vi "detectPulse.vi"(1 "filteredECG":waveform(dbl)) -> (0 "PulseBPM":dbl)   [LabVIEW 2023]
uses:
  <vilib>/measure/mamon.llb/Waveform Peak Detection for 1 Chan.vi
  <vilib>/measure/NI_MAPro.lvlib
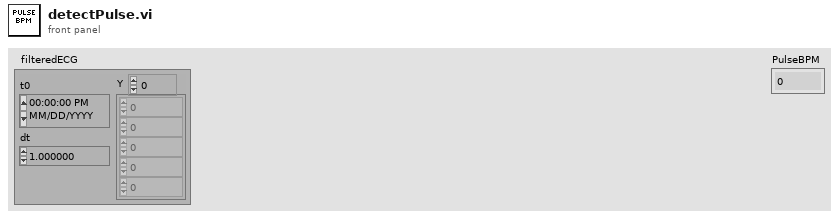
[diagram p1: front panel]
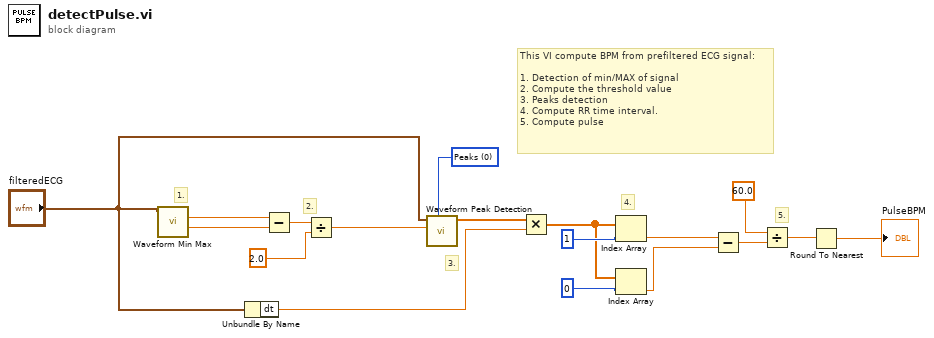
[diagram p0: block diagram]
diagram:
  w1 = u16 0 items=["Peaks", "Valleys"] ("peaks/valleys")
  # "5."
  # "This VI compute BPM from prefiltered ECG signal:\n\n1. Detection of min/MAX of signal\n2. Compute the threshold value\n3. Peaks detection\n4. Compute RR time interval.\n5. Compute pulse"
  # "4."
  # "3."
  # "2."
  # "1."
  n1 = call <vilib>:"Waveform Min Max.vi"("waveform in"="filteredECG") -> ("Y min"=w17:dbl, "Y max"=w18:dbl)  [unwired: 5 in, 4 out]
  n2 = Unbundle By Name("filteredECG") -> ("dt"=w12:dbl)
  n3 = Subtract(x=w18, y=w17) -> (x-y=w15:dbl)
  n4 = Divide(x=w15, y=2.0) -> (x/y=w14:dbl)
  n5 = call-poly <vilib>:"Waveform Peak Detection.vi"("peaks/valleys"=w1, "threshold"=w14, "Signal In"="filteredECG") -> ("Locations"=w11:dbl[])  [unwired: 4 in, 4 out]
  n6 = Multiply(x=w11, y=w12) -> (x*y=w8:dbl[])
  n7 = Index Array(array=w8, index=1) -> (element=w7:dbl)
  n8 = Index Array(array=w8, index=0) -> (element=w6:dbl)
  n9 = Subtract(x=w7, y=w6) -> (x-y=w5:dbl)
  n10 = Divide(x=60.0, y=w5) -> (x/y=w3:dbl)
  n11 = Round To Nearest(number=w3) -> (nearest integer value=→"PulseBPM":dbl)
